vi "Auth Extra.vi"(8 "error in (no error)":errorcluster, 10 "authextra in":string="{}", 11 "IAuthenticator in":refnum<class "IAuthenticator.lvclass">) -> (0 "error out":errorcluster, 2 "authextra":string caption="authextra out", 3 "IAuthenticator out":refnum<class "IAuthenticator.lvclass">)   [LabVIEW 2020, in "wamplv.lvlib" / "IAuthenticator.lvclass"]
uses:
  IAuthenticator.lvclass
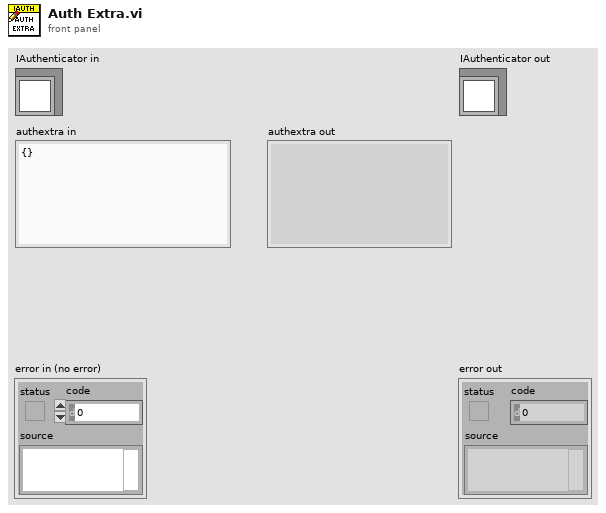
[diagram p1: front panel]
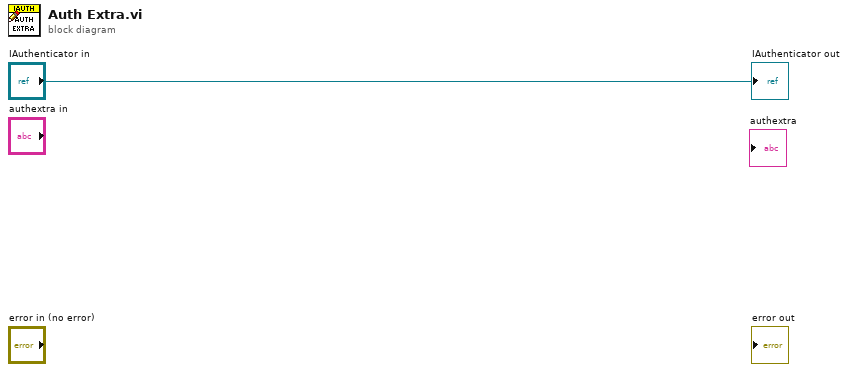
[diagram p0: block diagram]
diagram:
  "IAuthenticator out" <- "IAuthenticator in"
